vi "Pause.vi"(8 "error in":errorcluster, 11 "Elapsed Time":dbl) -> (0 "error out":errorcluster, 2 "New Elapsed Time":dbl, 3 "New Time Stamp":dbl)   [LabVIEW 2014]
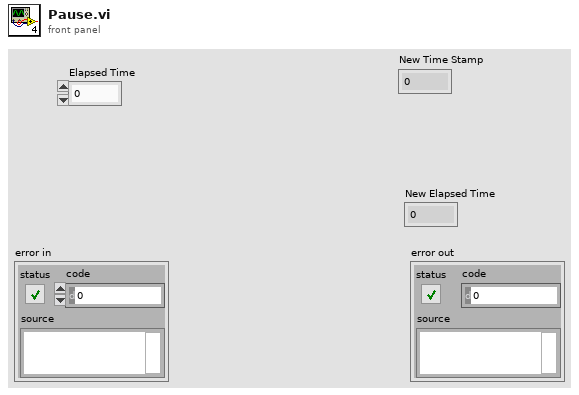
[diagram p1: front panel]
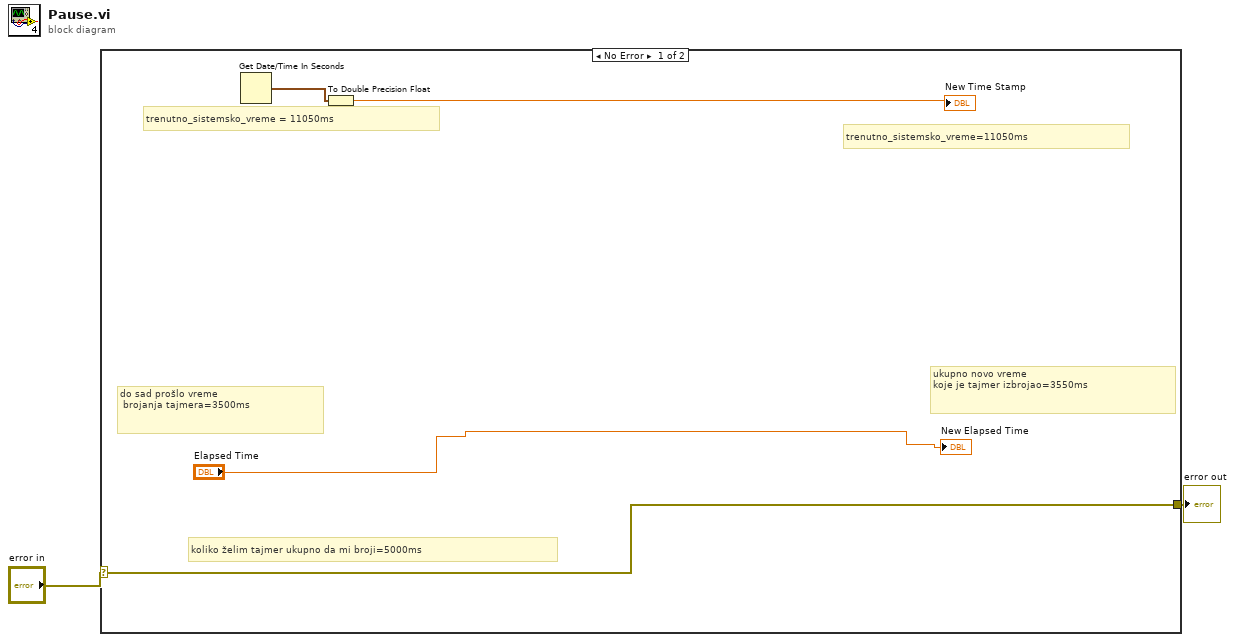
[diagram p0: block diagram]
diagram:
  n1 = case shown="No Error" "error in" {
    selector: "error in" -> [w4 w7]
    tunnel: [w4 w7] -> w1
    frame No Error {
      # "ukupno novo vreme \nkoje je tajmer izbrojao=3550ms"
      # "koliko želim tajmer ukupno da mi broji=5000ms"
      # "do sad prošlo vreme\n brojanja tajmera=3500ms"
      # "trenutno_sistemsko_vreme=11050ms"
      # "trenutno_sistemsko_vreme = 11050ms"
      n2 = Get Date/Time In Seconds() -> (seconds since 1Jan1904=w6:timestamp)
      n3 = To Double Precision Float(number=w6) -> (double precision float=→"New Time Stamp":dbl)
      "New Elapsed Time" <- "Elapsed Time"
    }
    frame Error {
    }
  }
  "error out" <- w1
